vi "+S2C_PCIe1762H_Process.vi"(8 "Error In":errorcluster) -> (0 "Error Out":errorcluster)   [LabVIEW 2024]
uses:
  VIs/S2C_PCIe1762H_Proc_Globals.vi
panel:
  out "Err":bool
  in  "Clear":bool
  out "Exit":bool
  in  "LogDepth":u32=10 caption="Log Depth"
  in  "CtrlTab":enum32{"PCIe1762H", "Read All DIO"}(tab)
  in  "P1":T1={"Init"={"Device"="DemoDevice", "Module Index"=0, "P1C1Exe"=FALSE}, "Digital Read"={"Foot Switch Read"=0, "ReadState"=FALSE, "P1C3Exe"=FALSE}, "Digital Write"={"Foot Switch Write"=0, "Write State"=FALSE, "P1C4Exe"=FALSE}, "Reset"={"P1C2Exe"=FALSE}} {"Digital Write"."Foot Switch Write" items=["Bipolar_FS", "LigCoag_FS", "LigBipolar_FS", "LigSeal_FS", "LigCut_FS", "LigSpare_FS", "Mono2Coag_FS", "Mono2Cut_FS", "Mono2VL_FS", "Mono2Spare_FS", "Mono1Coag_FS", "Mono1Cut_FS"]; "Digital Read"."Foot Switch Read" items=["Bipolar_FS", "LigCoag_FS", "LigBipolar_FS", "LigSeal_FS", "LigCut_FS", "LigSpare_FS", "Mono2Coag_FS", "Mono2Cut_FS", "Mono2VL_FS", "Mono2Spare_FS", "Mono1Coag_FS", "Mono1Cut_FS"]}
  in  "P2":T2
  in  "CommLog":string caption="Communication Log"
  # "Main Cluster:\n394x886\n1 = 355x876\n2 = 355x438\n3 = 355x292\n4 = 163x438\n6 = 163x292\n8 = 163x219"
  # "PCIe1762H Driver Panel"
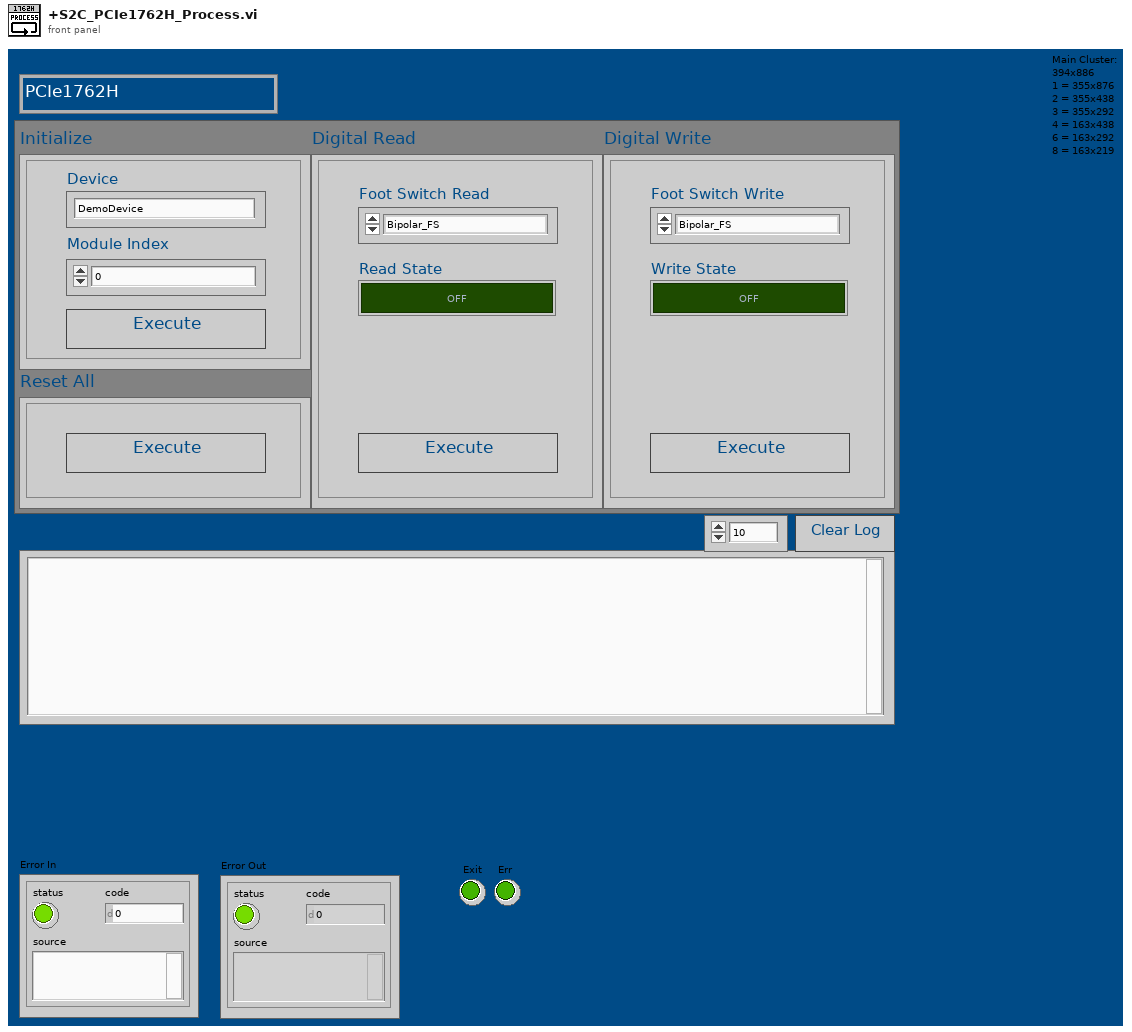
[diagram p1: front panel]
types:
  T1 = cluster{"Init":cluster{"Device":string, "Module Index":i32, "P1C1Exe":bool}, "Digital Read":cluster{"Foot Switch Read":u16, "ReadState":bool, "P1C3Exe":bool}, "Digital Write":cluster{"Foot Switch Write":u16, "Write State":bool, "P1C4Exe":bool}, "Reset":cluster{"P1C2Exe":bool}}
  T2 = cluster{"ReadAll":cluster{"P2C1Exe":bool, "Bipolar_FS":bool, "LigCut_FS":bool, "Mono2VL_FS":bool, "Spare1":bool, "LigCoag_FS":bool, "LigSpare_FS":bool, "Mono2Spare_FS":bool, "Spare2":bool, "LigBipolar_FS":bool, "Mono2Coag_FS":bool, "Mono1Coag_FS":bool, "Spare3":bool, "LigSeal_FS":bool, "Mono2Cut_FS":bool, "Mono1Cut_FS":bool, "Spare4":bool}}
  T3 = cluster{"Caller-Q":refnum<queue>, "Command":string, "Return":string, "Data":variant, "Timeout":dbl}
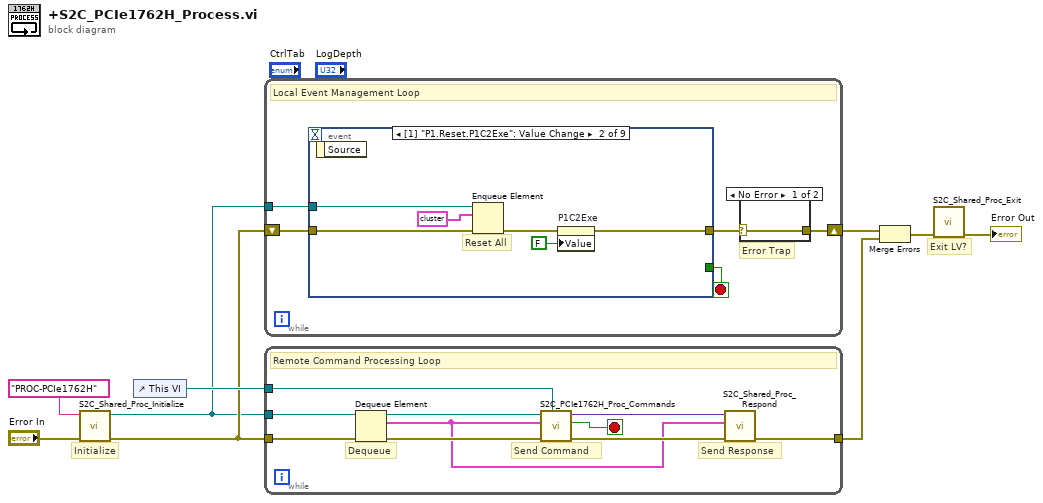
[diagram p0: block diagram]
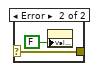
[diagram p2: hidden frame]
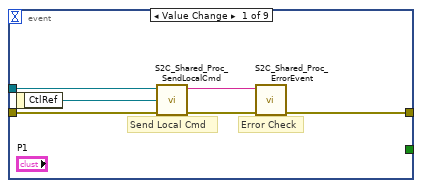
[diagram p3: hidden frame]
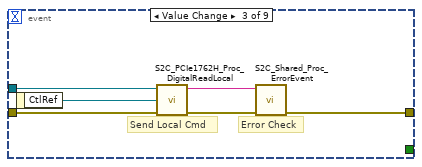
[diagram p4: hidden frame]
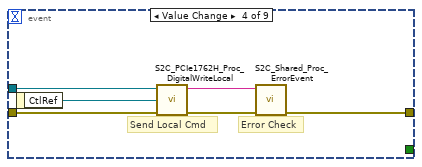
[diagram p5: hidden frame]
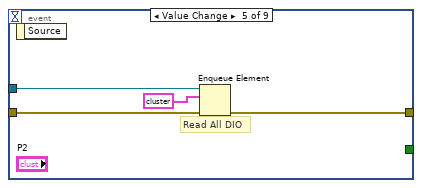
[diagram p6: hidden frame]
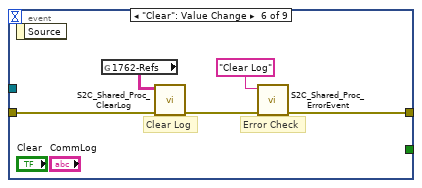
[diagram p7: hidden frame]
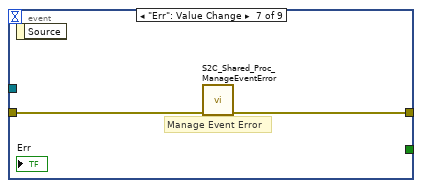
[diagram p8: hidden frame]
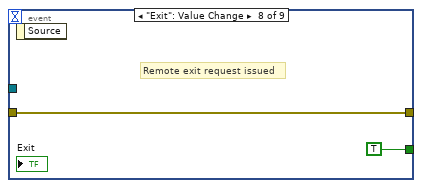
[diagram p9: hidden frame]
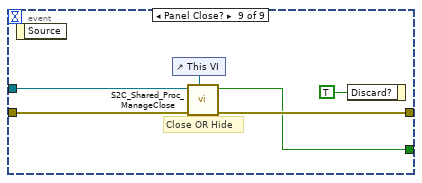
[diagram p10: hidden frame]
diagram:
  # "Exit LV?"
  # "Initialize"
  n1 = call "S2C_Shared_Proc_Initialize.vi"("Error In"="Error In", "Q-Name"="PROC-PCIe1762H" ("name (unnamed)")) -> ("Error Out"=w4:errorcluster, "Q-Ref"=w1:refnum<queue>)  [unwired: 8 in]
  n2 = control-ref of="This VI"() -> (w5:refnum<vi>)
  n3 = while {
    tunnel: w1 -> [w13]
    shift-right: [w10] -> w7
    shift-left: w4 -> [w14]
    stop <- w12 stop-if-true
    # "Error Trap"
    # "Local Event Management Loop"
    n4 = event shown="[1] \"P1.Reset.P1C2Exe\": Value Change" {
      selector: _ -> [_ _ _ _ _ _ _ _ _]
      dyn-events: _ -> [_ _ _ _ _ _ _ _ _]
      timeout: _ -> [_ _ _ _ _ _ _ _ _]
      tunnel: w14 -> [w23 w28 w35 w41 w45 w50 w52 w54 w59]
      tunnel: w13 -> [w22 w27 w34 w40 w44 _ _ _ w57]
      tunnel: [w19 w25 w31 w37 w43 w48 w51 w54 w58] -> w11
      tunnel: [_ _ _ _ _ _ _ TRUE ("Discard?") w56] -> w12
      event "P1.Init.P1C1Exe": Value Change {
        # "Error Check"
        # "Send Local Cmd"
        n5 = event-data() -> ("CtlRef"=w21:refnum<vi>)  [unwired: 1 in]
        n6 = call "S2C_Shared_Proc_SendLocalCmd.vi"("Error In"=w23, "ExeRef"=w21, "Q-Ref"=w22) -> ("Error Out"=w20:errorcluster, "Command"=w18:string)  [unwired: 7 in]
        n7 = call "S2C_Shared_Proc_ErrorEvent.vi"("Error In"=w20, "Command"=w18) -> ("Error Out"=w19:errorcluster)  [unwired: 9 in]
      }
      event "P1.Reset.P1C2Exe": Value Change {
        # "Reset All"
        n8 = event-data() -> ()  [unwired: 1 in, 1 out]
        n9 = Enqueue Element(queue=w27, element=T3 {"Caller-Q"=refnum, "Command"="^Reset All", "Return"="", "Data"=variant, "Timeout"=0.0}, error in (no error)=w28) -> (error out=w26:errorcluster)  [unwired: 1 in, 2 out]
        n10 = property on="P1C2Exe" class="Bool (strict)"(error in=w26, "Value"=FALSE) -> (error out=w25:errorcluster)  [unwired: 1 in, 1 out]
      }
      event "P1.Digital Read.P1C3Exe": Value Change {
        # "Error Check"
        # "Send Local Cmd"
        n11 = event-data() -> ("CtlRef"=w33:refnum<vi>)  [unwired: 1 in]
        n12 = call "S2C_PCIe1762H_Proc_DigitalReadLocal.vi"("Error In"=w35, "ExeRef"=w33, "Q-Ref"=w34) -> ("Error Out"=w32:errorcluster, "Command"=w30:string)  [unwired: 7 in]
        n13 = call "S2C_Shared_Proc_ErrorEvent.vi"("Error In"=w32, "Command"=w30) -> ("Error Out"=w31:errorcluster)  [unwired: 9 in]
      }
      event "P1.Digital Write.P1C4Exe": Value Change {
        # "Error Check"
        # "Send Local Cmd"
        n14 = event-data() -> ("CtlRef"=w39:refnum<vi>)  [unwired: 1 in]
        n15 = call "S2C_PCIe1762H_Proc_DigitalWriteLocal.vi"("Error In"=w41, "ExeRef"=w39, "Q-Ref"=w40) -> ("Error Out"=w38:errorcluster, "Command"=w36:string)  [unwired: 7 in]
        n16 = call "S2C_Shared_Proc_ErrorEvent.vi"("Error In"=w38, "Command"=w36) -> ("Error Out"=w37:errorcluster)  [unwired: 9 in]
      }
      event "P2.ReadAll.P2C1Exe": Value Change {
        # "Read All DIO"
        n17 = event-data() -> ()  [unwired: 1 in, 1 out]
        n18 = Enqueue Element(queue=w44, element=T3 {"Caller-Q"=refnum, "Command"="^Read All DIO", "Return"="", "Data"=variant, "Timeout"=0.0}, error in (no error)=w45) -> (error out=w43:errorcluster)  [unwired: 1 in, 2 out]
      }
      event "Clear": Value Change {
        # "Error Check"
        # "Clear Log"
        n19 = event-data() -> ()  [unwired: 1 in, 1 out]
        n20 = global read "S2C_PCIe1762H_Proc_Globals.vi" "1762-Refs"() -> (w46:string[][])
        n21 = call "S2C_Shared_Proc_ClearLog.vi"("Error In"=w50, "Refs"=w46) -> ("Error Out"=w49:errorcluster)  [unwired: 9 in]
        n22 = call "S2C_Shared_Proc_ErrorEvent.vi"("Error In"=w49, "Command"="Clear Log") -> ("Error Out"=w48:errorcluster)  [unwired: 9 in]
      }
      event "Err": Value Change {
        # "Manage Event Error"
        n23 = event-data() -> ()  [unwired: 1 in, 1 out]
        n24 = call "S2C_Shared_Proc_ManageEventError.vi"("Error In"=w52) -> ("Error Out"=w51:errorcluster)  [unwired: 10 in]
      }
      event "Exit": Value Change {
        # "Remote exit request issued"
        n25 = event-data() -> ()  [unwired: 1 in, 1 out]
      }
      event Panel Close? {
        # "Close OR Hide"
        n26 = event-data() -> ()  [unwired: 1 in, 1 out]
        n27 = control-ref of="This VI"() -> (w55:refnum<vi>)
        n28 = call "S2C_Shared_Proc_ManageClose.vi"("VI_Ref"=w55, "Error In"=w59, "Q-Ref"=w57) -> ("Error Out"=w58:errorcluster, "Exit?"=w56:bool)  [unwired: 7 in]
        n29 = event-data("Discard?"=TRUE) -> ()  [unwired: 1 in, 1 out]
      }
    }
    n30 = case shown="No Error" w11 {
      selector: w11 -> [w15 w17]
      tunnel: [w15 w17] -> w10
      frame No Error {
      }
      frame Error {
        n31 = property on="Err" class="Bool (strict)"("Val(Sgnl)"=FALSE ("Value (Signaling)")) -> ()  [unwired: 2 in, 2 out]
      }
    }
  }
  n32 = while {
    tunnel: w1 -> [w61]
    tunnel: w5 -> [w65]
    tunnel: w4 -> [w70]
    tunnel: [w64] -> w6
    stop <- w66 stop-if-true
    # "Send Response"
    # "Send Command"
    # "Dequeue"
    # "Remote Command Processing Loop"
    n33 = Dequeue Element(queue=w61, error in (no error)=w70) -> (queue out=w63:refnum<queue>, element=w62:T3, error out=w69:errorcluster)  [unwired: 1 in, 1 out]
    n34 = call "S2C_PCIe1762H_Proc_Commands.vi"("VI_Ref"=w65, "Error In"=w69, "Settings"=w62, "Q-Ref"=w63) -> ("Error Out"=w67:errorcluster, "Stop?"=w66:bool, "Response"=w68:variant)  [unwired: 5 in]
    n35 = call "S2C_Shared_Proc_Respond.vi"("Error In"=w67, "Settings"=w62, "Response"=w68) -> ("Error Out"=w64:errorcluster)  [unwired: 8 in]
  }
  n36 = Merge Errors(w7, w6) -> (w3:errorcluster)
  n37 = call "S2C_Shared_Proc_Exit.vi"("Error In"=w3) -> ("Error Out"=→"Error Out":errorcluster)  [unwired: 10 in]
